vi "Clear Hardware.vi"(2 "error in (no error)":errorcluster, 3 "Pulseblaster in":refnum<class "Pulseblaster.lvclass">) -> (0 "error out":errorcluster, 1 "Pulseblaster out":refnum<class "Pulseblaster.lvclass">)   [LabVIEW 2013, in "Pulseblaster.lvclass"]
uses:
  Pulseblaster.lvclass
  Utils_devs/SpinAPI/SpinAPI-20140801.lvlib
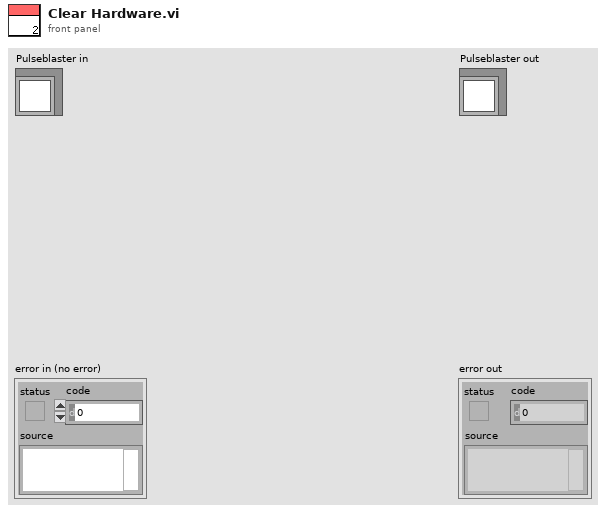
[diagram p1: front panel]
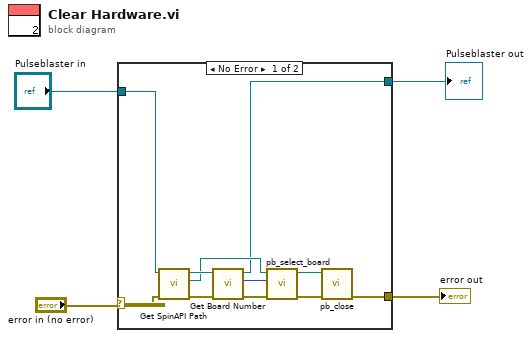
[diagram p0: block diagram]
diagram:
  n1 = case shown="No Error" "error in (no error)" {
    selector: "error in (no error)" -> [w6 w17]
    tunnel: [w5 w17] -> w3
    tunnel: "Pulseblaster in" -> [w8 w16]
    tunnel: [w7 w16] -> w1
    frame No Error {
      n2 = call-dynamic "Get SpinAPI Path.vi"("error in (no error)"=w6, "Pulseblaster in"=w8) -> ("error out"=w15:errorcluster, "SpinAPI Path"=w9:path, "Pulseblaster out"=w10:refnum<class "Pulseblaster.lvclass">)  [unwired: 7 in]
      n3 = call-dynamic "Get Board Number.vi"("error in (no error)"=w15, "Pulseblaster in"=w10) -> ("error out"=w14:errorcluster, "Board Number"=w11:i32, "Pulseblaster out"=w7:refnum<class "Pulseblaster.lvclass">)  [unwired: 7 in]
      n4 = call "pb_select_board.vi"("error in (no error)"=w14, "board_num"=w11, "path in"=w9) -> ("error out"=w13:errorcluster, "path out"=w12:path)  [unwired: 7 in]
      n5 = call "pb_close.vi"("error in (no error)"=w13, "path in"=w12) -> ("error out"=w5:errorcluster)  [unwired: 8 in, 1 out]
    }
    frame Error {
    }
  }
  "error out" <- w3
  "Pulseblaster out" <- w1
